vi "Mapa Global.vi"() -> ()   [LabVIEW 2014]
panel:
  out "Mapa":cluster{dbl[], dbl[]}(graph)
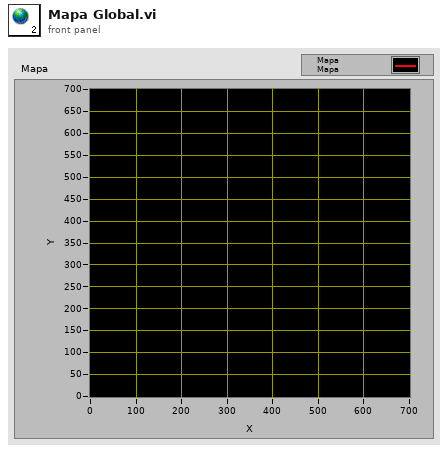
[diagram p1: front panel]
diagram:
